vi "Write Report Path.vi"(8 "error in (no error)":errorcluster, 10 "Report Path":path, 11 "csv-formatter in":refnum<class "csv-formatter.lvclass">) -> (0 "error out":errorcluster, 3 "csv-formatter out":refnum<class "csv-formatter.lvclass">)   [LabVIEW 2015, in "csv-formatter.lvclass"]
uses:
  csv-formatter.lvclass
  csv-formatter.lvclass/csv-formatter.ctl
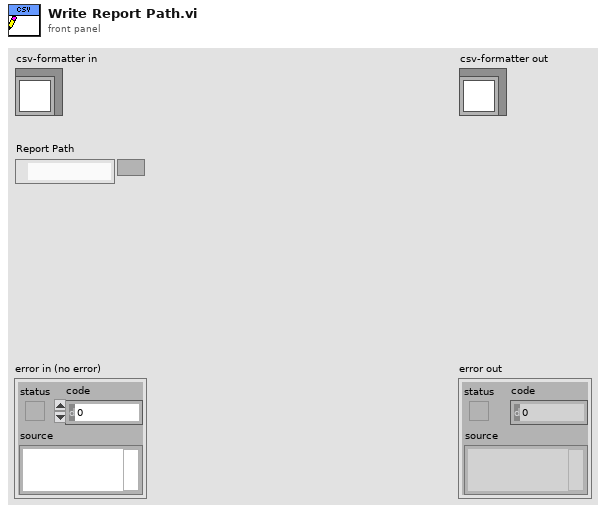
[diagram p1: front panel]
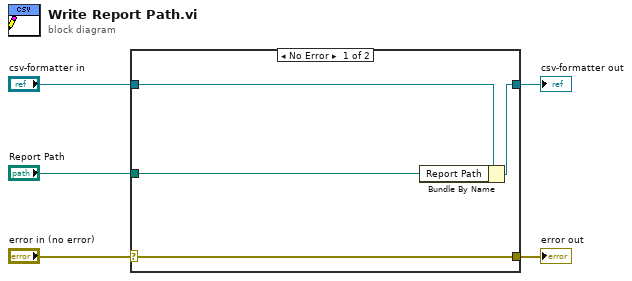
[diagram p0: block diagram]
diagram:
  n1 = case shown="No Error" "error in (no error)" {
    selector: "error in (no error)" -> [w9 w10]
    tunnel: [w9 w10] -> w4
    tunnel: [w7 w11] -> w2
    tunnel: "csv-formatter in" -> [w8 w11]
    tunnel: "Report Path" -> [w6 _]
    frame No Error {
      n2 = Bundle By Name(cluster=w8, "Report Path"=w6) -> (w7:refnum<class "csv-formatter.lvclass">)
    }
    frame Error {
    }
  }
  "error out" <- w4
  "csv-formatter out" <- w2
